vi "Write Configuration (INI) File.vi"   [LabVIEW 2016]
doc: "Illustrates how to create and write a configuration settings file. Enter values in the controls on the front panel then click on the Run Arrow. To read the file, run Read Configuration (INI) File.vi."
uses:
  <vilib>/Utility/config.llb/Write Key (Boolean).vi
  <vilib>/Utility/config.llb/Write Key (Double).vi
  <vilib>/Utility/config.llb/Write Key (Path).vi
  <vilib>/Utility/config.llb/Write Key (String).vi
  <vilib>/Utility/config.llb/NI_LVConfig.lvlib
panel:
  # "Overview: Demonstrates the use of the Configuration File VIs to write data to a configuration (INI) file.\nInstructions:\n1. Run this VI.\n2. Open Read Configuration (INI) File.vi and follow the instructions on its front panel."
types:
  T1 = typedef "NI_LVConfig.lvlib/Config Data RefNum.ctl" = refnum<k1>
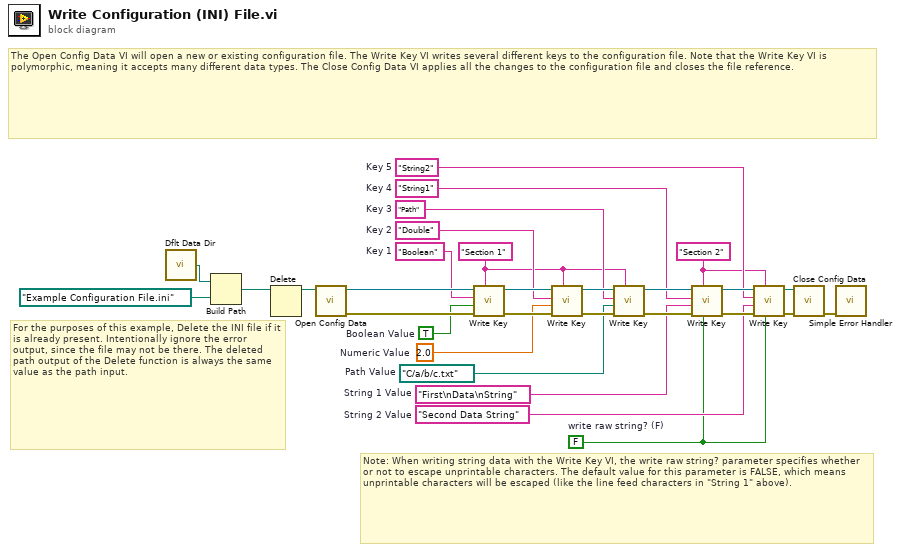
[diagram p0: block diagram]
diagram:
  w12 = "Second Data String"  # String 2 Value
  w13 = "First\nData\nString"  # String 1 Value
  w8 = path "C:/a/b/c.txt"  # Path Value
  w7 = 2.0  # Numeric Value
  w6 = TRUE  # Boolean Value
  w1 = FALSE  # write raw string? (F)
  w14 = "String2"  # Key 5
  w15 = "String1"  # Key 4
  w16 = "Path"  # Key 3
  w17 = "Double"  # Key 2
  w18 = "Boolean"  # Key 1
  w9 = "Section 2"
  w10 = "Section 1"
  # "Note: When writing string data with the Write Key VI, the write raw string? parameter specifies whether or not to escape unprintable characters. The default value for this parameter is FALSE, which means unprintable characters will be escaped (like the line feed characters in \"String 1\" above)."
  # "The Open Config Data VI will open a new or existing configuration file. The Write Key VI writes several different keys to the configuration file. Note that the Write Key VI is polymorphic, meaning it accepts many different data types. The Close Config Data VI applies all the changes to the configuration file and closes the file reference."
  # "For the purposes of this example, Delete the INI file if it is already present. Intentionally ignore the error output, since the file may not be there. The deleted path output of the Delete function is always the same value as the path input."
  n1 = call <vilib>:"Dflt Data Dir.vi"() -> ("App:Default Data Directory"=w4:path)
  n2 = Build Path(base path=w4, name or relative path=path "Example Configuration File.ini" ("default name")) -> (appended path=w2:path)
  n3 = Delete(path (use dialog)=w2) -> (deleted path=w3:path)  [unwired: 4 in, 2 out]
  n4 = call <vilib>:"Open Config Data.vi"("configuration file path"=w3) -> ("error out"=w24:errorcluster, "refnum"=w30:T1)  [unwired: 2 in, 7 out]
  n5 = call-poly <vilib>:"Write Key.vi"("section"=w10, "error in (no error)"=w24, "value"=w6, "key"=w18, "refnum"=w30) -> ("error out"=w23:errorcluster, "refnum out"=w29:T1)  [unwired: 5 out]
  n6 = call-poly <vilib>:"Write Key.vi"("section"=w10, "error in (no error)"=w23, "value"=w7, "key"=w17, "refnum"=w29) -> ("error out"=w22:errorcluster, "refnum out"=w28:T1)  [unwired: 3 in, 2 out]
  n7 = call-poly <vilib>:"Write Key.vi"("section"=w10, "error in (no error)"=w22, "value"=w8, "key"=w16, "refnum"=w28) -> ("error out"=w21:errorcluster, "refnum out"=w27:T1)  [unwired: 5 out]
  n8 = call-poly <vilib>:"Write Key.vi"("write raw string? (F)"=w1, "section"=w9, "error in (no error)"=w21, "value"=w13, "key"=w15, "refnum"=w27) -> ("error out"=w20:errorcluster, "refnum out"=w26:T1)  [unwired: 4 out]
  n9 = call-poly <vilib>:"Write Key.vi"("write raw string? (F)"=w1, "section"=w9, "error in (no error)"=w20, "value"=w12, "key"=w14, "refnum"=w26) -> ("error out"=w19:errorcluster, "refnum out"=w25:T1)  [unwired: 4 out]
  n10 = call <vilib>:"Close Config Data.vi"("error in (no error)"=w19, "refnum"=w25) -> ("error out"=w11:errorcluster)  [unwired: 1 in, 8 out]
  n11 = call <vilib>:"Simple Error Handler.vi"("error in (no error)"=w11) -> ()  [unwired: 1 in, 8 out]
